vi "ReleaseDC.vi"(8 "error in (no error)":errorcluster, 10 "hdc":u32, 11 "hWnd":u32) -> (0 "error out":errorcluster, 3 "return":u32)   [LabVIEW 2019]
uses:
  user32.dll
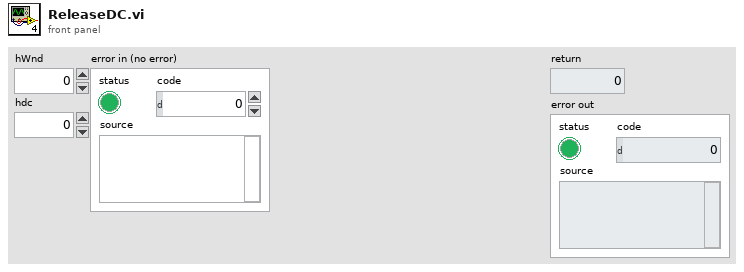
[diagram p1: front panel]
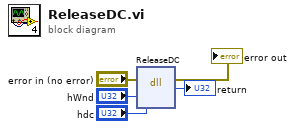
[diagram p0: block diagram]
diagram:
  n1 = dll-call lib="user32.dll" fn="ReleaseDC" label="GetDC"(error in="error in (no error)", "hWnd"="hWnd", "hdc"="hdc") -> (error out=→"error out":errorcluster, "return"=→"return":u32)  [unwired: 4 in, 1 out]
